vi "License - Password.vi"(8 "error in":errorcluster) -> (0 "error out":errorcluster, 2 "T button?":bool, 3 "Pass?":bool)   [LabVIEW 2019]
panel:
  in  "Button":bool
  in  "Password":string
  # "Please Keyin Password"
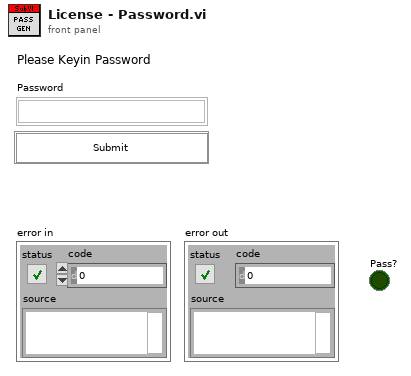
[diagram p1: front panel]
types:
  T1 = typedef "eventvkey.ctl" = enum16{"ASCII", "Enter", "Return", "Shift", "Ctrl", "Alt", "Cmd", "Opt", "Caps", "NumLock", "Clear", "Break", "Up", "Down", "Left", "Right", "Insert", "Delete", "Home", "End", "PageUp", "PageDown", "Escape", "Help", "Pause", "ScrollLock", "F1", "F2", "F3", "F4", "F5", "F6", "F7", "F8", "F9", "F10", "F11", "F12", "F13", "F14", "F15", "F16", "F17", "F18", "F19", "F20", "F21", "F22", "F23", "F24", "Play", "VolumeUp", "VolumeDown", "Mute", "Two Byte Char"}
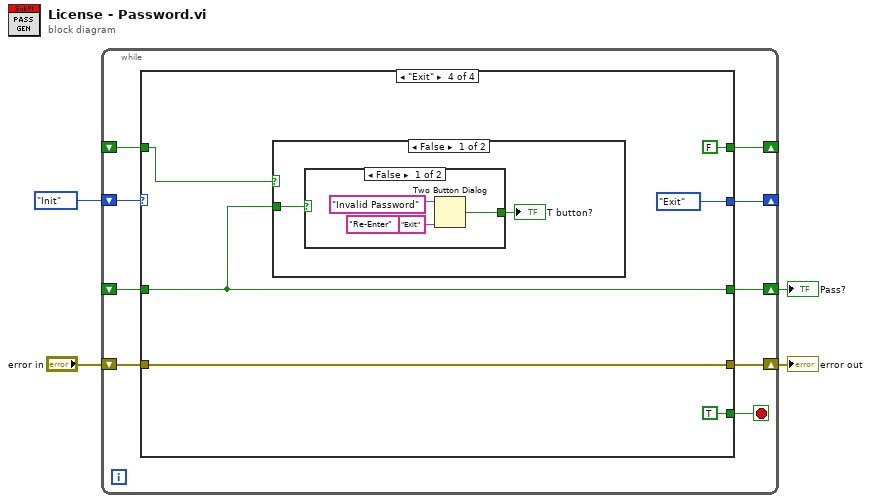
[diagram p0: block diagram]
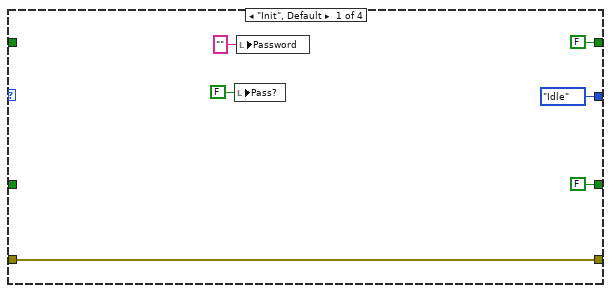
[diagram p2: hidden frame]
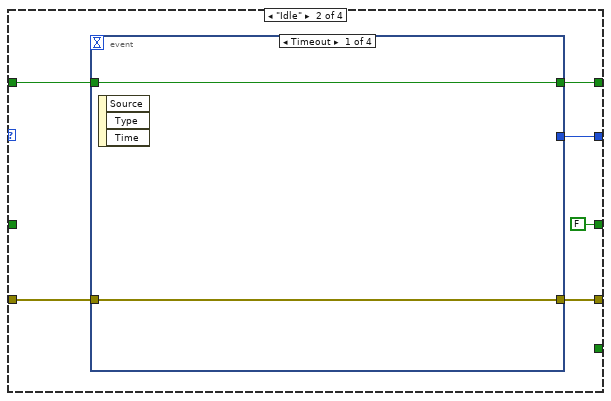
[diagram p3: hidden frame]
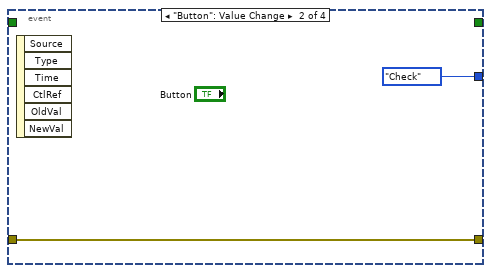
[diagram p4: hidden frame]
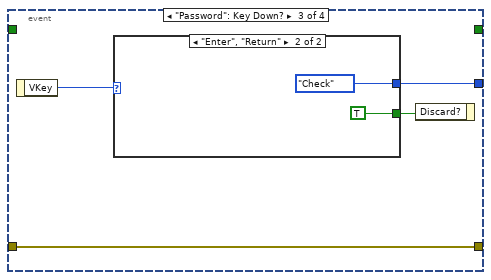
[diagram p5: hidden frame]
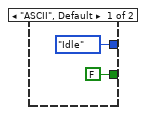
[diagram p6: hidden frame]
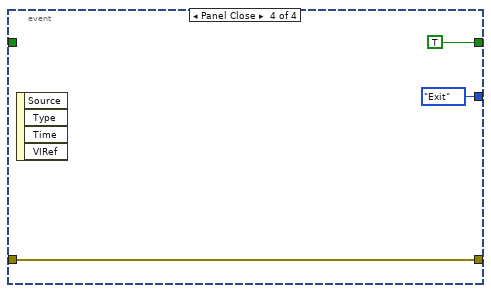
[diagram p7: hidden frame]
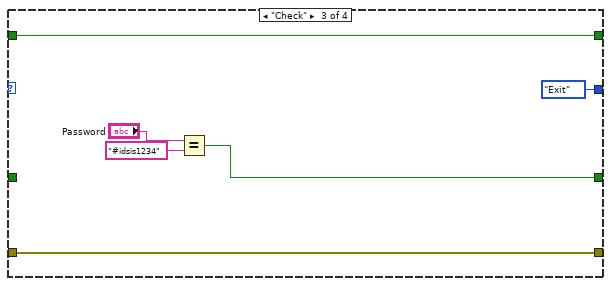
[diagram p8: hidden frame]
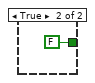
[diagram p9: hidden frame]
diagram:
  n1 = while {
    shift-right: [w12] -> _
    shift-left: enum16{"Init", "Idle", "Check", "Exit"}."Init" -> [w13]
    shift-right: [w11] -> w3
    shift-left: _ -> [w10]
    shift-right: [w8] -> w1
    shift-left: "error in" -> [w7]
    shift-right: [w6] -> _
    shift-left: _ -> [w5]
    stop <- w9 stop-if-true
    n2 = case shown="\"Exit\"" w13 {
      tunnel: [enum16{"Init", "Idle", "Check", "Exit"}."Idle" w25 enum16{"Init", "Idle", "Check", "Exit"}."Exit" enum16{"Init", "Idle", "Check", "Exit"}."Exit" ("f")] -> w12
      tunnel: [FALSE FALSE w42 w51] -> w11
      tunnel: w10 -> [_ _ _ w51]
      tunnel: [_ _ _ TRUE] -> w9
      tunnel: [w15 w23 w43 w52] -> w8
      tunnel: w7 -> [w15 w22 w43 w52]
      tunnel: [FALSE w21 w41 FALSE] -> w6
      tunnel: w5 -> [_ w20 w41 w50]
      frame "Init", Default {
        n3 = local write "Pass?"(FALSE ("Pass?")) -> ()
        n4 = local write "Password"("" ("Password")) -> ()
      }
      frame "Idle" {
        n5 = event shown="[0] Timeout" {
          selector: _ -> [_ _ _ _]
          dyn-events: _ -> [_ _ _ _]
          timeout: _ -> [_ _ _ _]
          tunnel: [_ enum16{"Init", "Idle", "Check", "Exit"}."Check" w32 enum16{"Init", "Idle", "Check", "Exit"}."Exit"] -> w25
          tunnel: [w27 w28 w30 w40] -> w23
          tunnel: w22 -> [w27 w28 w30 w40]
          tunnel: [w26 _ _ TRUE] -> w21
          tunnel: w20 -> [w26 _ _ _]
          event Timeout {
            n6 = event-data() -> ()  [unwired: 1 in, 3 out]
          }
          event "Button": Value Change {
            n7 = event-data() -> ()  [unwired: 1 in, 6 out]
          }
          event "Password": Key Down? {
            n8 = event-data() -> ("VKey"=w33:T1)  [unwired: 1 in]
            n9 = case shown="\"Enter\", \"Return\"" w33 {
              tunnel: [enum16{"Init", "Idle", "Check", "Exit"}."Idle" enum16{"Init", "Idle", "Check", "Exit"}."Check"] -> w32
              tunnel: [FALSE TRUE] -> w31
              frame "ASCII", Default {
              }
              frame "Enter", "Return" {
              }
            }
            n10 = event-data("Discard?"=w31) -> ()  [unwired: 1 in, 1 out]
          }
          event Panel Close {
            n11 = event-data() -> ()  [unwired: 1 in, 4 out]
          }
        }
      }
      frame "Check" {
        n12 = Equal?(x="Password", y="#idsis1234") -> (x = y?=w42:bool)
      }
      frame "Exit" {
        n13 = case shown="False" w50 {
          tunnel: w51 -> [w54 _]
          frame False {
            n14 = case shown="False" w54 {
              tunnel: [w56 FALSE ("T button?")] -> w53
              frame False {
                n15 = Two Button Dialog(message="Invalid Password", 1:"Exit" ("F button name (\"Cancel\")"), 2:"Re-Enter" ("T button name (\"OK\")")) -> (T button?=w56:bool)
              }
              frame True {
              }
            }
            "T button?" <- w53
          }
          frame True {
          }
        }
      }
    }
  }
  "Pass?" <- w3
  "error out" <- w1
